vi "Read Sensor Input Status Register.vi"(8 "error in (no error)":errorcluster, 11 "CAP1208 in":refnum<class "CAP1208.lvclass">) -> (0 "error out":errorcluster, 1 "Sensor Input (U8)":u8, 2 "Sensor Input (CS1-CS8)":bool[](array[boolean]), 3 "CAP1208 out":refnum<class "CAP1208.lvclass">)   [LabVIEW 2020, in "CAP1208.lvclass"]
uses:
  CAP1208.lvclass
  CAP1208.lvclass/CAP1208.ctl
  Read I2C.vi
  Write I2C.vi
  LINX I2C/LINX I2C.lvclass
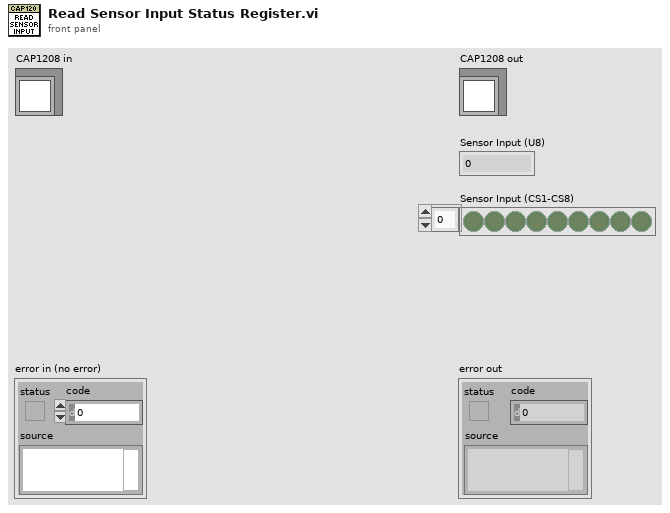
[diagram p1: front panel]
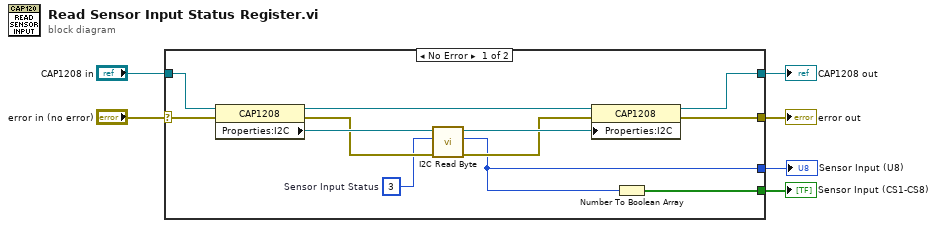
[diagram p0: block diagram]
diagram:
  n1 = case shown="No Error" "error in (no error)" {
    selector: "error in (no error)" -> [w10 w20]
    tunnel: [w13 w20] -> w5
    tunnel: [w12 w19] -> w3
    tunnel: "CAP1208 in" -> [w18 w19]
    tunnel: [w8 _] -> w2
    tunnel: [w7 _] -> w1
    frame No Error {
      w9 = u8 3  # Sensor Input Status
      n2 = property class="CAP1208"(reference=w18, error in=w10) -> (reference out=w11:refnum<class "CAP1208.lvclass">, error out=w15:errorcluster, "Properties:I2C"=w17:refnum<class "LINX I2C.lvclass">)
      n3 = call-dynamic "I2C Read Byte.vi"("error in (no error)"=w15, "Register Address"=w9, "LINX I2C in"=w17) -> ("error out"=w14:errorcluster, "Byte Read"=w7:u8, "LINX I2C out"=w16:refnum<class "LINX I2C.lvclass">)  [unwired: 6 in]
      n4 = property class="CAP1208"(reference=w11, error in=w14, "Properties:I2C"=w16) -> (reference out=w12:refnum<class "CAP1208.lvclass">, error out=w13:errorcluster)
      n5 = Number To Boolean Array(number=w7) -> (Boolean array=w8:bool[])
    }
    frame Error {
    }
  }
  "error out" <- w5
  "CAP1208 out" <- w3
  "Sensor Input (CS1-CS8)" <- w2
  "Sensor Input (U8)" <- w1
